vi "Get Dealt Player Name and Cards.vi"(11 "Hand History String in":string) -> (1 "Dealt Cards":string, 2 "Dealt Player Name":string, 3 "Hand History String Out":string)   [LabVIEW 2021]
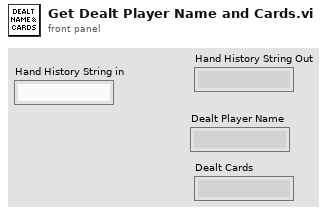
[diagram p1: front panel]
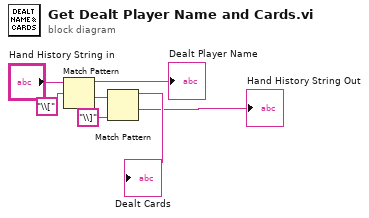
[diagram p0: block diagram]
diagram:
  n1 = Match Pattern(string="Hand History String in", regular expression="\\[") -> (before substring=→"Dealt Player Name":string, after substring=w4:string)  [unwired: 1 in, 2 out]
  n2 = Match Pattern(string=w4, regular expression="\\]") -> (before substring=→"Dealt Cards":string, after substring=→"Hand History String Out":string)  [unwired: 1 in, 2 out]
